vi "Camera_Mean_OCR_recheck.vi"(0 "Image Path":path=path "C:/images/img1.jpeg", 1 "Ctl Refnum":refnum<vi>, 9 "Filter Type":T3(ring)=enum."Differentiation", 11 "error in (no error)":errorcluster, 12 "Filtered image":T2=refnum) -> (3 "OCR Check":T1, 4 "OCR Recheck":bool, 6 "Mean Value Max":sgl=4.1535125 format="%.2f", 8 "Image Dst Out":T2, 10 "Curent Mean Value":sgl=4.1535125 format="%.2f", 13 "Image out":T2(plugin-control), 15 "error out":errorcluster)   [LabVIEW 2019]
uses:
  <vilib>/vision/Image Controls.llb/IMAQ Image.ctl
  <vilib>/vision/NI_Vision_Development_Module.lvlib
panel:
  out "Pattern Presence":bool=TRUE
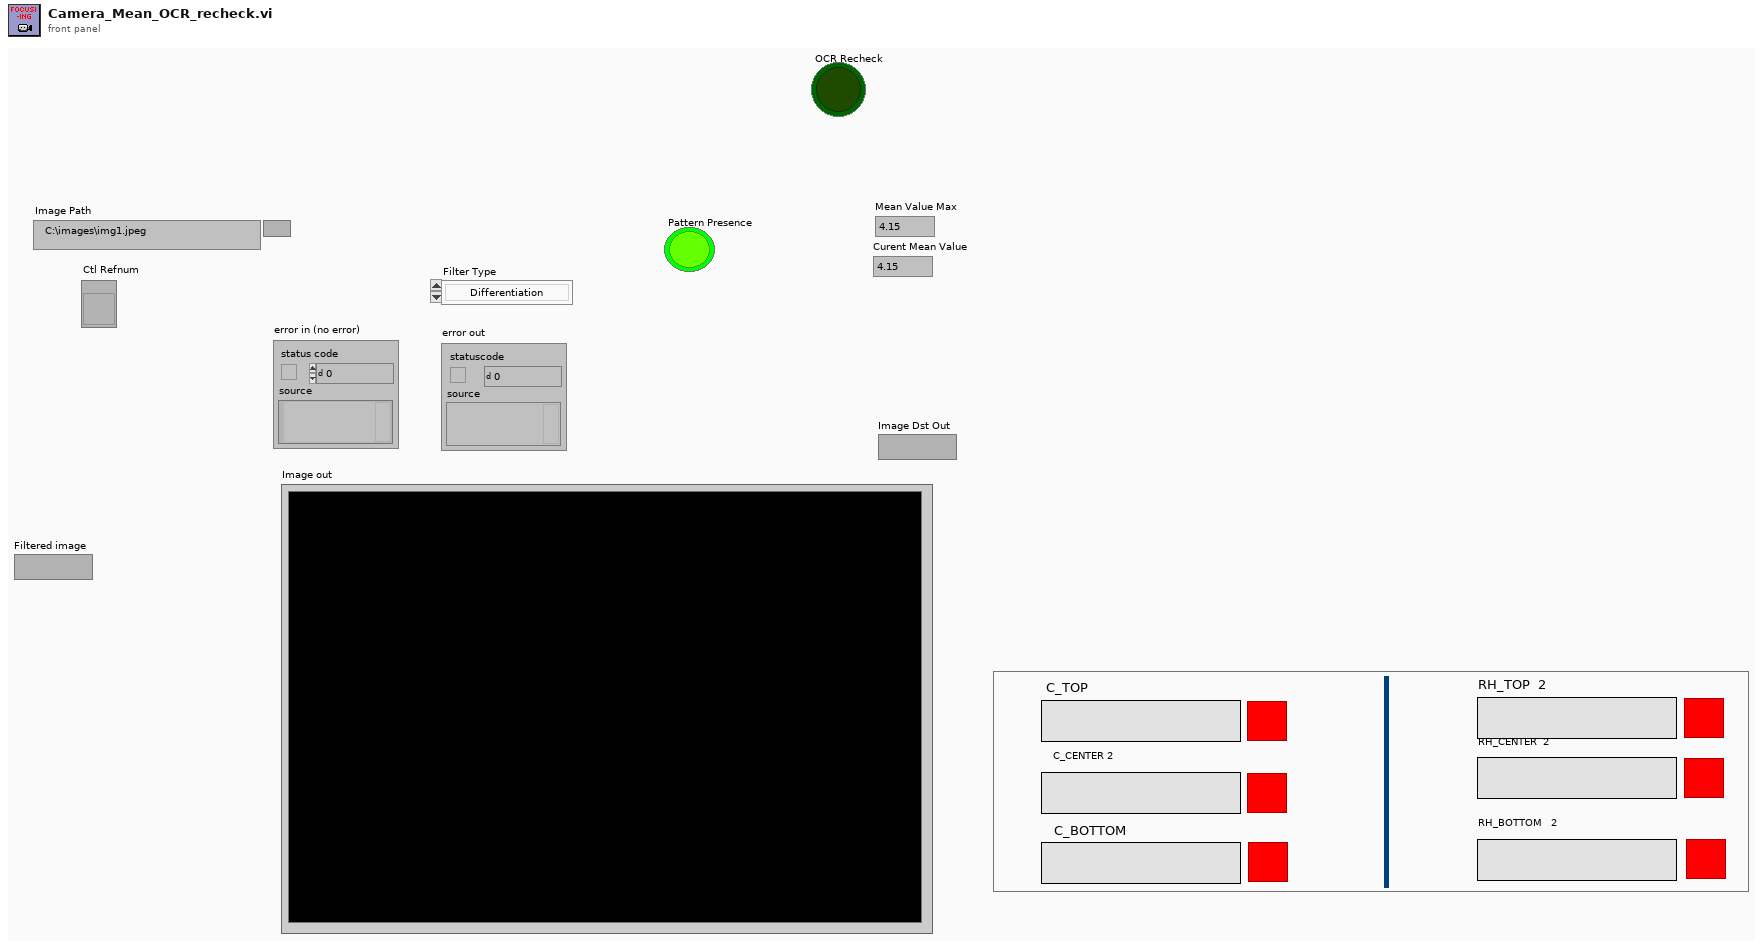
[diagram p1: front panel]
types:
  T1 = cluster{"RH_BOTTOM":bool, "RH_CENTER":bool, "RH_TOP":bool, "BOTTOM":bool, "CENTER":bool, "TOP":bool, "RH_BOTTOM   2":string, "RH_CENTER  2":string, "RH_TOP  2":string, "C_BOTTOM ":string, "C_CENTER 2":string, "C_TOP":string}
  T2 = typedef "IMAQ Image.ctl" = refnum<image>
  T3 = enum16{"Convolution", "Differentiation", "Gradient", "Prewitt", "Roberts", "Sigma", "Sobel"}
  T4 = typedef "Image Type" = u32
  T5 = enum32{"Differentiation", "Gradient", "Prewitt", "Roberts", "Sigma", "Sobel"}
  T6 = cluster{"C_Center":string, "Center 2":bool, "C_Top":string, "Top 2":bool, "C_Bottom":string, "Bottom 2":bool, "RH_TOP":string, "Top_RH":bool, "RH_CENTER":string, "Center_RH":bool, "RH_BOTTOM":string, "Bottom_RH":bool}
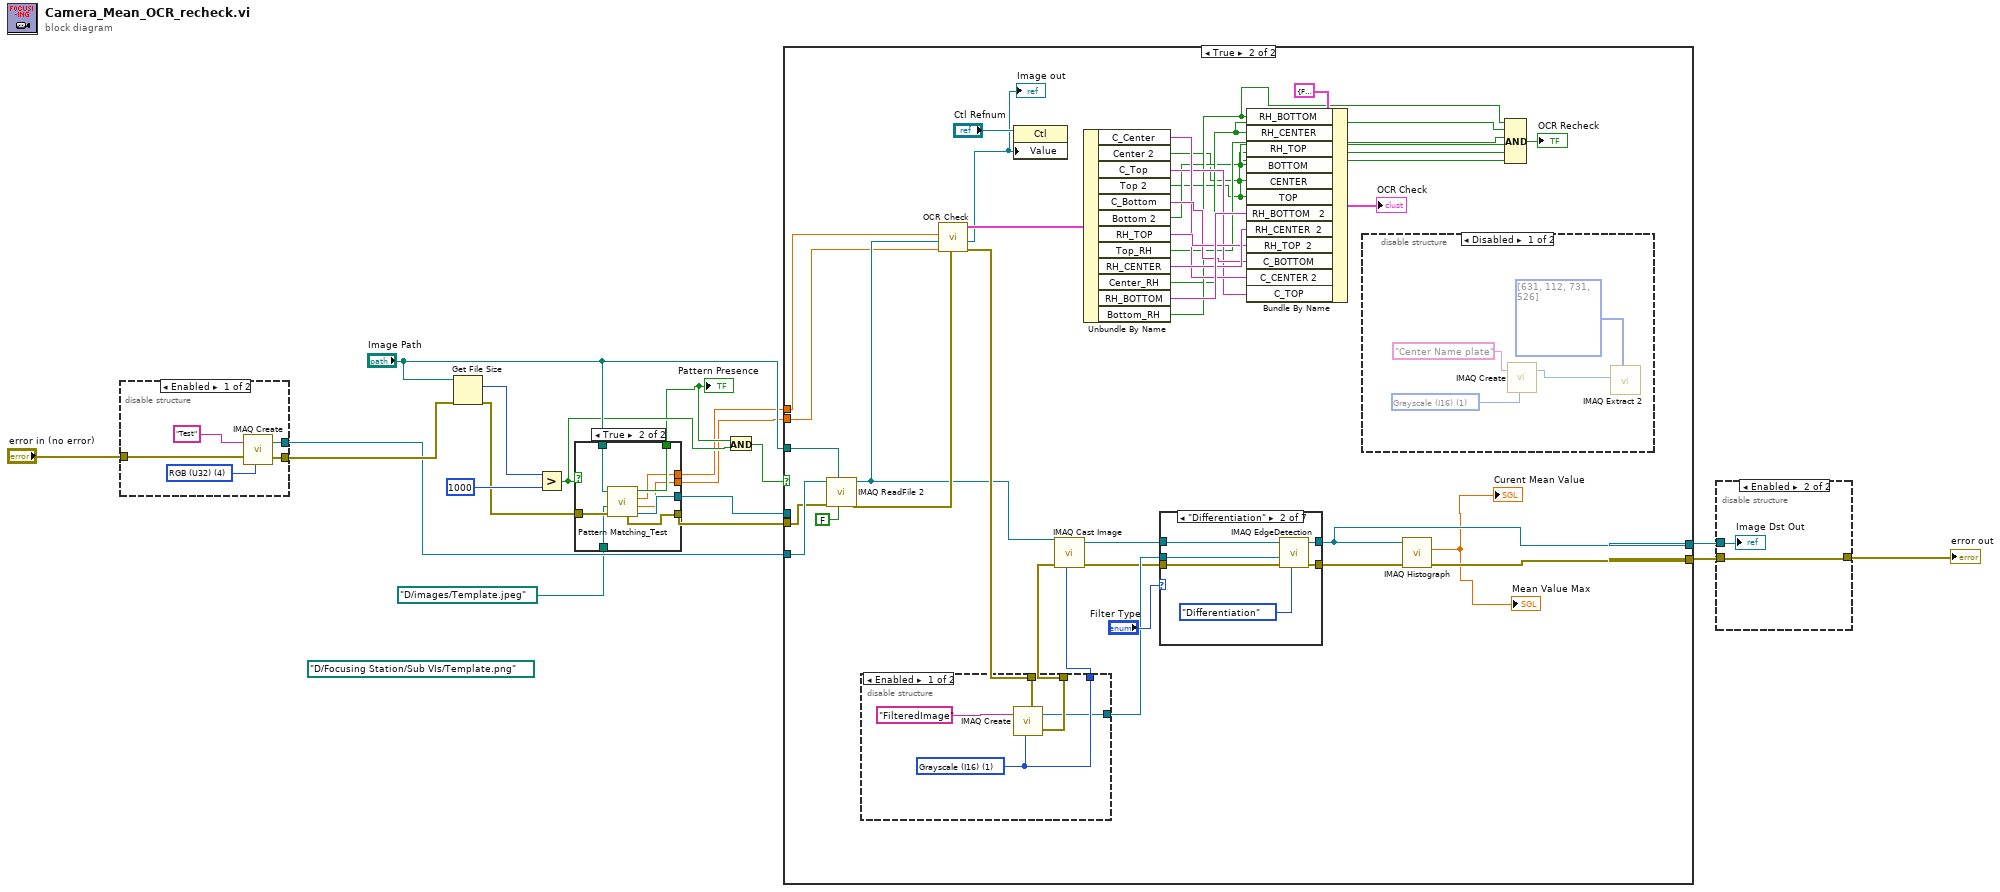
[diagram p0: block diagram]
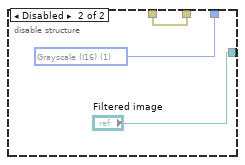
[diagram p6: hidden frame]
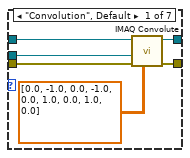
[diagram p7: hidden frame]
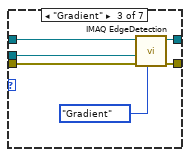
[diagram p8: hidden frame]
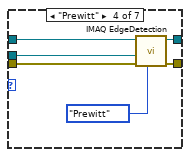
[diagram p9: hidden frame]
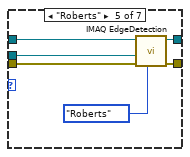
[diagram p10: hidden frame]
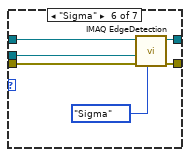
[diagram p11: hidden frame]
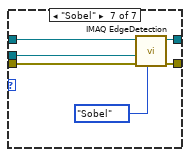
[diagram p12: hidden frame]
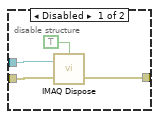
[diagram p13: hidden frame]
diagram:
  (unwired) path "D:/Focusing Station/Sub VIs/Template.png" ("Image File Path")
  n1 = disable-structure shown="Enabled" {
    disable-tunnel: [w21 w24] -> w12
    disable-tunnel: [w20 _] -> w11
    disable-tunnel: "error in (no error)" -> [w19 w24]
    frame Enabled {
      w22 = T4 4 items=["Grayscale (U8)", "Grayscale (I16)", "Grayscale (SGL)", "Complex (CSG)", "RGB (U32)", "HSL (U32)", "RGB (U64)", "Grayscale (U16)"] ("Image Type")
      n2 = call "IMAQ Create"("Image Name"="Test", "Image Type"=w22, "error in (no error)"=w19) -> ("New Image"=w20:T2, "error out"=w21:errorcluster)  [unwired: 2 in]
    }
    frame Disabled {
    }
  }
  n3 = Get File Size(file="Image Path", error in=w12) -> (size (in bytes)=w14:i64, 0:w10:errorcluster)  [unwired: 1 out]
  n4 = Greater?(x=w14, y=i64 1000) -> (0:w7:bool)
  n5 = case shown="True" w7 {
    tunnel: "Image Path" -> [_ w33]
    tunnel: w10 -> [w25 w32]
    tunnel: [_ w31] -> w9
    tunnel: [_ w30] -> w5
    tunnel: [w25 w29] -> w8
    tunnel: [_ w28] -> w4
    tunnel: [_ w27] -> w3
    tunnel: path "D:/images/Template.jpeg" ("Image File Path") -> [_ w26]
    frame False {
    }
    frame True {
      n6 = call "Pattern Matching_Test.vi"("error in (no error)"=w32, "Template file path"=w26, "File Path"=w33) -> ("Image out"=w31:T2, "y"=w27:sgl, "x"=w28:sgl, "Pattern Presence"=w30:bool, "error out"=w29:errorcluster)  [unwired: 4 in]
    }
  }
  "Pattern Presence" <- w5
  n7 = And(x=w5, y=w7) -> (x .and. y?=w6:bool)
  n8 = case shown="True" w6 {
    tunnel: "Image Path" -> [_ w61]
    tunnel: w11 -> [w35 w66]
    tunnel: [w34 w65] -> w18
    tunnel: [w35 w64] -> w17
    tunnel: w9 -> [_ _]
    tunnel: w8 -> [w34 w62]
    tunnel: w4 -> [_ w47]
    tunnel: w3 -> [_ w46]
    frame False {
    }
    frame True {
      n9 = call "IMAQ ReadFile 2"("Use File Path Image Type"=FALSE, "File Path"=w61, "error in (no error)"=w62, "Image"=w66) -> ("error out"=w51:errorcluster, "Image Out"=w50:T2)  [unwired: 3 in, 3 out]
      n10 = call "OCR Check.vi"("error in"=w51, "y"=w46, "Image in"=w50, "x"=w47) -> ("error out"=w52:errorcluster, "Image Out"=w48:T2, "OCR Check"=w49:T6)  [unwired: 4 in, 1 out]
      "Image out" <- w48
      n11 = disable-structure shown="Enabled" {
        disable-tunnel: w52 -> [w81 w84]
        disable-tunnel: [w79 w84] -> w71
        disable-tunnel: [w78 w82] -> w70
        disable-tunnel: [w77 "Filtered image"] -> w68
        frame Enabled {
          w78 = T4 1 items=["Grayscale (U8)", "Grayscale (I16)", "Grayscale (SGL)", "Complex (CSG)", "RGB (U32)", "HSL (U32)", "RGB (U64)", "Grayscale (U16)"] ("Image Type")
          n12 = call "IMAQ Create"("Image Name"="FilteredImage", "Image Type"=w78, "error in (no error)"=w81) -> ("New Image"=w77:T2, "error out"=w79:errorcluster)  [unwired: 2 in]
        }
        frame Disabled {
          w82 = T4 1 items=["Grayscale (U8)", "Grayscale (I16)", "Grayscale (SGL)", "Complex (CSG)", "RGB (U32)", "HSL (U32)", "RGB (U64)", "Grayscale (U16)"] ("Image Type")
        }
      }
      n13 = property class="Ctl"(reference="Ctl Refnum", "Value"=w48) -> ()  [unwired: 1 in, 2 out]
      n14 = call "IMAQ Cast Image"("Image Type"=w70, "error in (no error)"=w71, "Image Src"=w50) -> ("error out"=w37:errorcluster, "Image Dst Out"=w36:T2)  [unwired: 7 in]
      n15 = Unbundle By Name(w49) -> ("C_Center"=w54:string, "Center 2"=w41:bool, "C_Top"=w53:string, "Top 2"=w40:bool, "C_Bottom"=w55:string, "Bottom 2"=w42:bool, "RH_TOP"=w56:string, "Top_RH"=w43:bool, "RH_CENTER"=w57:string, "Center_RH"=w44:bool, "RH_BOTTOM"=w58:string, "Bottom_RH"=w45:bool)
      n16 = case shown="\"Differentiation\"" "Filter Type" {
        tunnel: w36 -> [w89 w95 w101 w107 w113 w119 w125]
        tunnel: w37 -> [w88 w94 w100 w106 w112 w118 w124]
        tunnel: w68 -> [w87 w96 w102 w108 w114 w120 w126]
        tunnel: [w86 w91 w97 w103 w109 w115 w121] -> w67
        tunnel: [w85 w92 w98 w104 w110 w116 w122] -> w64
        frame "Convolution", Default {
          n17 = call "IMAQ Convolute"("Kernel"=sgl[][] [[0.0, -1.0, 0.0], [-1.0, 0.0, 1.0], [0.0, 1.0, 0.0]], "error in (no error)"=w88, "Image Dst"=w87, "Image Src"=w89) -> ("error out"=w86:errorcluster, "Image Dst Out"=w85:T2)  [unwired: 6 in]
        }
        frame "Differentiation" {
          n18 = call "IMAQ EdgeDetection"("Method"=T5."Differentiation", "error in (no error)"=w94, "Image Dst"=w96, "Image Src"=w95) -> ("error out"=w91:errorcluster, "Image Dst Out"=w92:T2)  [unwired: 6 in]
        }
        frame "Gradient" {
          n19 = call "IMAQ EdgeDetection"("Method"=T5."Gradient", "error in (no error)"=w100, "Image Dst"=w102, "Image Src"=w101) -> ("error out"=w97:errorcluster, "Image Dst Out"=w98:T2)  [unwired: 6 in]
        }
        frame "Prewitt" {
          n20 = call "IMAQ EdgeDetection"("Method"=T5."Prewitt", "error in (no error)"=w106, "Image Dst"=w108, "Image Src"=w107) -> ("error out"=w103:errorcluster, "Image Dst Out"=w104:T2)  [unwired: 6 in]
        }
        frame "Roberts" {
          n21 = call "IMAQ EdgeDetection"("Method"=T5."Roberts", "error in (no error)"=w112, "Image Dst"=w114, "Image Src"=w113) -> ("error out"=w109:errorcluster, "Image Dst Out"=w110:T2)  [unwired: 6 in]
        }
        frame "Sigma" {
          n22 = call "IMAQ EdgeDetection"("Method"=T5."Sigma", "error in (no error)"=w118, "Image Dst"=w120, "Image Src"=w119) -> ("error out"=w115:errorcluster, "Image Dst Out"=w116:T2)  [unwired: 6 in]
        }
        frame "Sobel" {
          n23 = call "IMAQ EdgeDetection"("Method"=T5."Sobel", "error in (no error)"=w124, "Image Dst"=w126, "Image Src"=w125) -> ("error out"=w121:errorcluster, "Image Dst Out"=w122:T2)  [unwired: 6 in]
        }
      }
      n24 = Bundle By Name(cluster=T1 {"RH_BOTTOM"=FALSE, "RH_CENTER"=FALSE, "RH_TOP"=FALSE, "BOTTOM"=FALSE, "CENTER"=FALSE, "TOP"=FALSE, "RH_BOTTOM   2"="", "RH_CENTER  2"="", "RH_TOP  2"="", "C_BOTTOM "="", "C_CENTER 2"="", "C_TOP"=""} ("OCR Check"), "RH_BOTTOM"=w45, "RH_CENTER"=w44, "RH_TOP"=w43, "BOTTOM"=w42, "CENTER"=w41, "TOP"=w40, "RH_BOTTOM   2"=w58, "RH_CENTER  2"=w57, "RH_TOP  2"=w56, "C_BOTTOM"=w55, "C_CENTER 2"=w54, "C_TOP"=w53) -> (→"OCR Check":T1)
      n25 = disable-structure shown="Disabled" {
        frame Disabled {
          w76 = T4 1 items=["Grayscale (U8)", "Grayscale (I16)", "Grayscale (SGL)", "Complex (CSG)", "RGB (U32)", "HSL (U32)", "RGB (U64)", "Grayscale (U16)"] ("Image Type")
          n26 = call "IMAQ Create"("Image Name"="Center Name plate", "Image Type"=w76) -> ("New Image"=w74:T2)  [unwired: 3 in, 1 out]
          n27 = call "IMAQ Extract 2"("Optional Rectangle"=i32[] [631, 112, 731, 526], "Image Dst"=w74) -> ()  [unwired: 8 in, 2 out]
        }
        frame Enabled {
        }
      }
      n28 = call "IMAQ Histograph"("error in (no error)"=w67, "Image"=w64) -> ("error out"=w65:errorcluster, "Mean Value"=→"Curent Mean Value" →"Mean Value Max":sgl)  [unwired: 6 in, 2 out]
      n29 = Compound Arithmetic op=AND(w45, w44, w43, w42, w41, w40) -> (→"OCR Recheck":bool)
    }
  }
  n30 = disable-structure shown="Enabled" {
    disable-tunnel: w18 -> [w130 w132]
    disable-tunnel: w17 -> [w129 w131]
    disable-tunnel: [w127 w132] -> w16
    frame Disabled {
      n31 = call "IMAQ Dispose"("All Images? (No)"=TRUE, "Image"=w129, "error in (no error)"=w130) -> ("error out"=w127:errorcluster)  [unwired: 3 in]
    }
    frame Enabled {
      "Image Dst Out" <- w131
    }
  }
  "error out" <- w16
